vi "Configure Channel.vi"(8 "error in (no error)":errorcluster, 9 "Config Channel":T1={"Channel (0: Channel 1)"=0, "Vertical Coupling (1: DC)"=1, "Probe Attenuation (10: 10X)"=10, "Vertical Range (10.0 V/div)"=10.0, "Vertical Offset (0.0 divs)"=0.0, "Bandwidth (0: MAX Bandwidth)"=0, "Enable Channel (True)"=TRUE} {"Bandwidth (0: MAX Bandwidth)" items=["MAX Bandwidth", "Unlimited"]; "Probe Attenuation (10: 10X)" items=["1"=1, "10"=10, "20"=20, "50"=50, "100"=100, "500"=500, "1000"=1000]; "Vertical Coupling (1: DC)" items=["AC", "DC", "Ground"]; "Channel (0: Channel 1)" items=["Channel 1", "Channel 2", "Channel 3", "Channel 4", "Math", "Reference A", "Reference B", "Reference C", "Reference D"]}, 11 "Osciloscope in":refnum<class "Osciloscope.lvclass">) -> (0 "error out":errorcluster, 3 "Osciloscope out":refnum<class "Osciloscope.lvclass">)   [LabVIEW 2020, in "Controlador.lvlib" / "Osciloscope.lvclass"]
uses:
  Osciloscope.lvclass
  Osciloscope.lvclass/Osciloscope.ctl
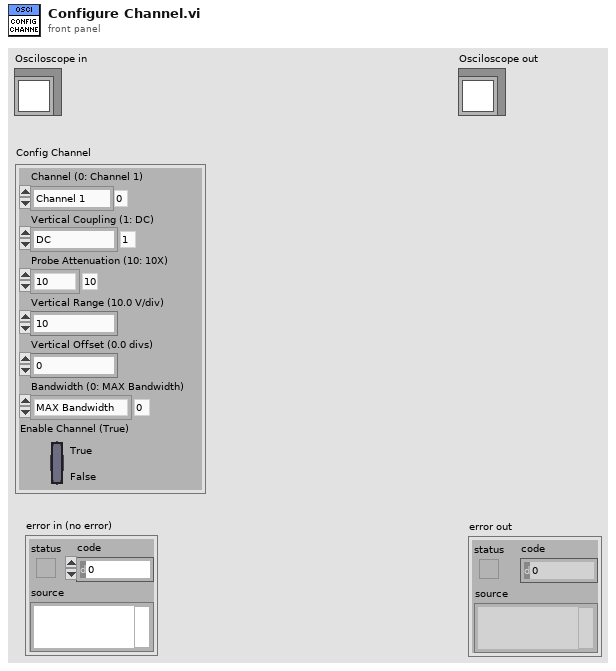
[diagram p1: front panel]
types:
  T1 = cluster{"Channel (0: Channel 1)":i32, "Vertical Coupling (1: DC)":i32, "Probe Attenuation (10: 10X)":i32, "Vertical Range (10.0 V/div)":dbl, "Vertical Offset (0.0 divs)":dbl, "Bandwidth (0: MAX Bandwidth)":i32, "Enable Channel (True)":bool}
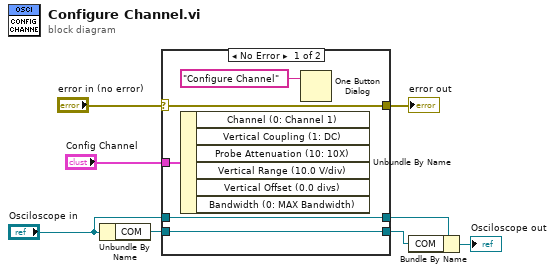
[diagram p0: block diagram]
diagram:
  n1 = Unbundle By Name("Osciloscope in") -> ("COM"=w4:refnum<visa-resource-name>)
  n2 = case shown="No Error" "error in (no error)" {
    selector: "error in (no error)" -> [w12 w15]
    tunnel: [w12 w15] -> w7
    tunnel: [w13 w14] -> w3
    tunnel: "Osciloscope in" -> [w13 w14]
    tunnel: [w11 _] -> w1
    tunnel: w4 -> [w11 _]
    tunnel: "Config Channel" -> [w10 _]
    frame No Error {
      n3 = Unbundle By Name(w10) -> ()  [unwired: 6 out]
      n4 = One Button Dialog(message="Configure Channel") -> ()  [unwired: 1 in, 1 out]
    }
    frame Error {
    }
  }
  "error out" <- w7
  n5 = Bundle By Name(cluster=w3, "COM"=w1) -> (→"Osciloscope out":refnum<class "Osciloscope.lvclass">)
